vi "실습 8-2 글로벌 변수02.vi"() -> ()   [LabVIEW 2014]
panel:
  out "웨이브폼 차트":dbl(graph)
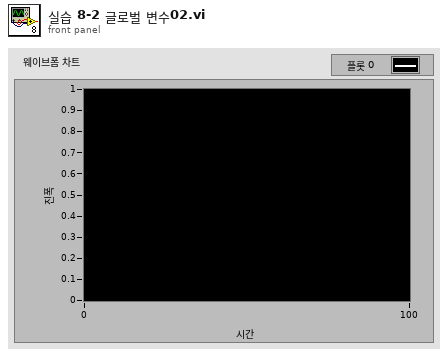
[diagram p1: front panel]
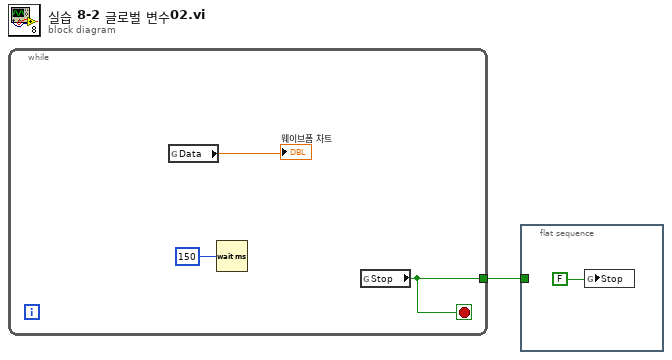
[diagram p0: block diagram]
diagram:
  n1 = while {
    tunnel: [w2] -> w1
    stop <- w2 stop-if-true
    n2 = global read "my글로벌.vi" "Data"() -> (→"웨이브폼 차트":dbl)
    n3 = Wait (ms)(milliseconds to wait=u32 150 ("대기 시간(ms)")) -> ()  [unwired: 1 out]
    n4 = global read "my글로벌.vi" "Stop"() -> (w2:bool)
  }
  n5 = flat-sequence {
    tunnel: w1 -> [_]
    frame #0 {
      n6 = global write "my글로벌.vi" "Stop"(FALSE) -> ()
    }
  }
